vi "Write elements.vi"(8 "error in (no error)":errorcluster, 10 "elements":refnum<class "Element.lvclass">[](array[class]), 11 "Topic in":refnum<class "Topic.lvclass">) -> (0 "error out":errorcluster, 3 "Topic out":refnum<class "Topic.lvclass">)   [LabVIEW 2018, in "Topic.lvclass"]
doc: "Write the elements."
uses:
  Topic.lvclass
  Element/Element.lvclass
  Topic.lvclass/Topic.ctl
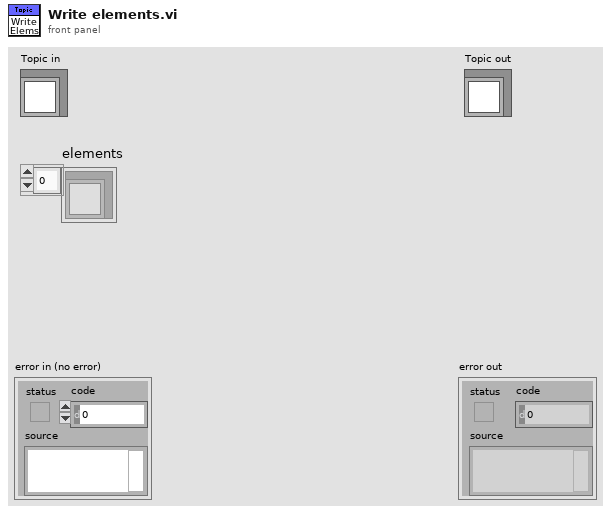
[diagram p1: front panel]
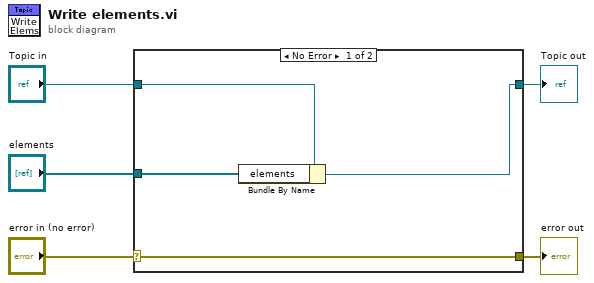
[diagram p0: block diagram]
diagram:
  n1 = case shown="No Error" "error in (no error)" {
    selector: "error in (no error)" -> [w9 w10]
    tunnel: [w9 w10] -> w4
    tunnel: [w7 w11] -> w2
    tunnel: "Topic in" -> [w8 w11]
    tunnel: "elements" -> [w6 _]
    frame No Error {
      n2 = Bundle By Name(cluster=w8, "elements"=w6) -> (w7:refnum<class "Topic.lvclass">)
    }
    frame Error {
    }
  }
  "error out" <- w4
  "Topic out" <- w2
